vi "DeleteDataFlowStep.vi"(8 "error in (no error)":errorcluster, 10 "type":T1, 11 "Dataflow step":string) -> (0 "error out":errorcluster)   [LabVIEW 2017, in "DataFlow.lvlib"]
doc: "Removes a process from the Dataflow Script."
uses:
  <vilib>/addons/InsightCM/Devices/Shared/Common/DataFlow/DataFlow.lvlib
  <vilib>/addons/InsightCM/Devices/Shared/Common/DataFlow/controls/Type.ctl
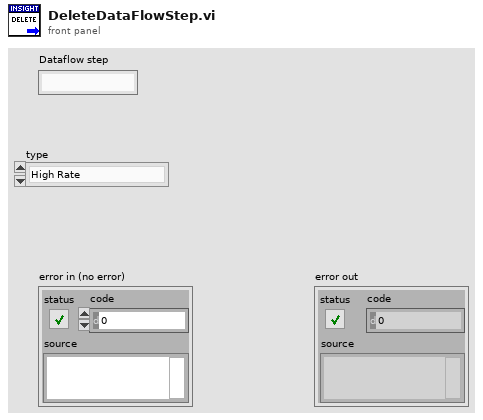
[diagram p1: front panel]
types:
  T1 = typedef "DataFlow.lvlib/Type.ctl" = enum16{"High Rate", "Low Rate", "Burst Mode"}
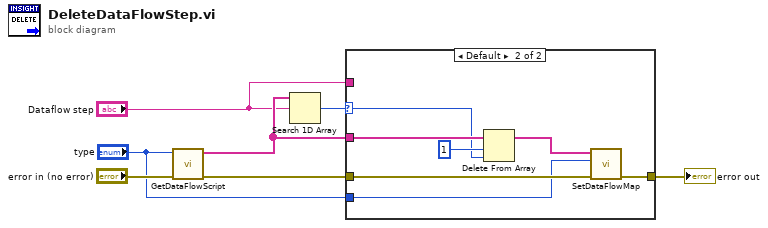
[diagram p0: block diagram]
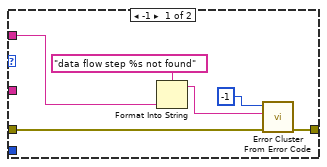
[diagram p2: hidden frame]
diagram:
  n1 = call <vilib>:"GetDataFlowScript.vi"("error in (no error)"="error in (no error)", "type"="type") -> ("error out"=w4:errorcluster, "Dataflow script"=w5:string[])  [unwired: 7 in, 1 out]
  n2 = Search 1D Array(1D array=w5, element="Dataflow step") -> (index of element=w6:i32)  [unwired: 1 in]
  n3 = case shown="Default" w6 {
    selector: w6 -> [_ w18]
    tunnel: w5 -> [_ w20]
    tunnel: w4 -> [w13 w17]
    tunnel: [w12 w16] -> w2
    tunnel: "Dataflow step" -> [w10 _]
    tunnel: "type" -> [_ w14]
    frame -1 {
      n4 = Format Into String(format string="data flow step %s not found", w10) -> (resulting string=w9:string)  [unwired: 2 in, 1 out]
      n5 = call <vilib>:"Error Cluster From Error Code.vi"("error in (no error)"=w13, "error message (\"\")"=w9, "error code (0)"=-1) -> ("error out"=w12:errorcluster)  [unwired: 6 in]
    }
    frame Default {
      n6 = Delete From Array(array=w20, length=1, index=w18) -> (array with subset deleted=w15:string[])  [unwired: 1 out]
      n7 = call <vilib>:"SetDataFlowMap.vi"("error in (no error)"=w17, "type"=w14, "Dataflow script"=w15) -> ("error out"=w16:errorcluster)  [unwired: 8 in]
    }
  }
  "error out" <- w2
